vi "TCP PC.vi"() -> ()   [LabVIEW 2011]
panel:
  in  "远程端口或服务名称":u16
  in  "地址":string
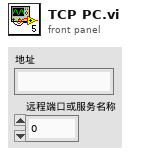
[diagram p1: front panel]
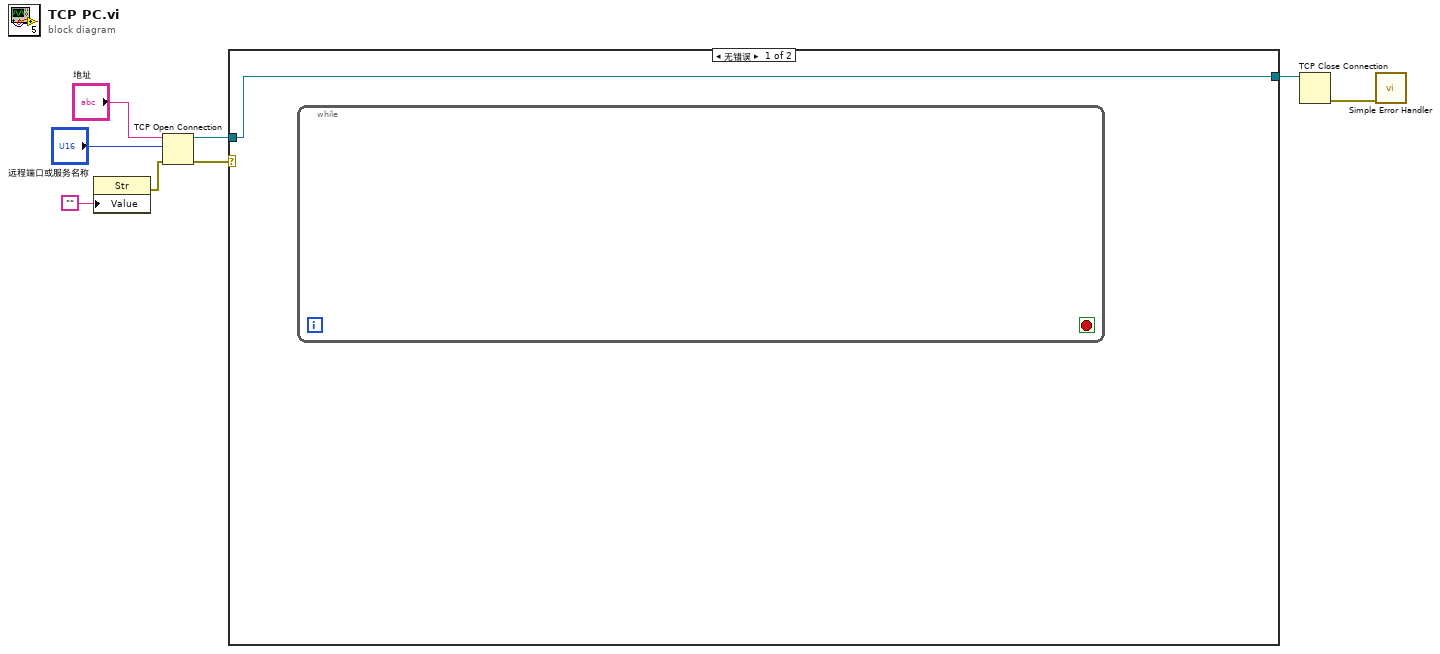
[diagram p0: block diagram]
diagram:
  n1 = property on="属性节点" class="Str"("Value"="") -> (error out=w5:errorcluster)  [unwired: 2 in, 1 out]
  n2 = TCP Open Connection(address="地址", remote port or service name="远程端口或服务名称", error in (no error)=w5) -> (connection ID=w3:refnum<k5>, error out=w8:errorcluster)  [unwired: 2 in]
  n3 = case shown="无错误" w8 {
    tunnel: w3 -> [w9 _]
    tunnel: [w9 _] -> w2
    frame No Error {
      n4 = while {
        stop <- _ stop-if-true
      }
    }
    frame Error {
    }
  }
  n5 = TCP Close Connection(connection ID=w2) -> (error out=w1:errorcluster)  [unwired: 2 in, 1 out]
  n6 = call <vilib>:"Simple Error Handler.vi"("error in (no error)"=w1) -> ()  [unwired: 4 in, 5 out]
